vi "Alpha Transparency and Z-Order.vi"() -> ()   [LabVIEW 2011]
uses:
  <vilib>/Heliosphere Research LLC/Advanced Plotting Toolkit/Advanced Plotting Toolkit.lvlib
  <vilib>/Heliosphere Research LLC/Advanced Plotting Toolkit/api_plotting/Histogram_Automatic.vi
  <vilib>/Heliosphere Research LLC/Advanced Plotting Toolkit/api_plotting/HistogramRange.ctl
  <vilib>/Heliosphere Research LLC/Advanced Plotting Toolkit/typedefs/PlotColor.ctl
  <vilib>/Heliosphere Research LLC/Advanced Plotting Toolkit/properties/Line_Style.ctl
  <vilib>/Heliosphere Research LLC/Advanced Plotting Toolkit/properties/Line.ctl
  <vilib>/Heliosphere Research LLC/Advanced Plotting Toolkit/properties/Display.ctl
  <vilib>/Heliosphere Research LLC/Advanced Plotting Toolkit/api_plotting/HistogramProperties.ctl
  <vilib>/Heliosphere Research LLC/Advanced Plotting Toolkit/properties/Text_FontSize.ctl
  <vilib>/Heliosphere Research LLC/Advanced Plotting Toolkit/properties/Text_FontStyle.ctl
  <vilib>/Heliosphere Research LLC/Advanced Plotting Toolkit/properties/Text.ctl
  <vilib>/Heliosphere Research LLC/Advanced Plotting Toolkit/api_annotations/TextProperties.ctl
panel:
  in  "Show Text":bool
  in  "Text Z-Order":dbl
  in  "Histogram Alpha":dbl=0.6
  out "Alpha Demo":picture
  # "Alpha Transparency and Z-Order"
  # "Most plotting VIs in the tookit have a Display sub-cluster\nin the property cluster.  This allows you to adjust how the\nobjects are rendered.\n\nWhen multiple plotting VIs are called, the objects are \"stacked\"\naccording to their Z-order.  This number is automatically\nassigned by the Toolkit and keeps e.g. text in front of bars and\nlines.  You can manually adjust the Z order to force objects\nto be displayed in front of or behind other objects.  Try it\nbelow; turn the sample text on and adjust its Z-Order.\n\nNormally, objects are opaque.  However, you can enable\ntransparency using the Display.Alpha value.  This value ranges\nfrom 0 (fully transparent) to 1 (fully opaque).  Traditional\nalpha-blending is used, which can combine multiple partially-\ntransparent objects along with the plot background color.\n\nIn this example, two histogram plots are made, and their\nalpha values set to 0.6. Try changing this value and see the\nresults."
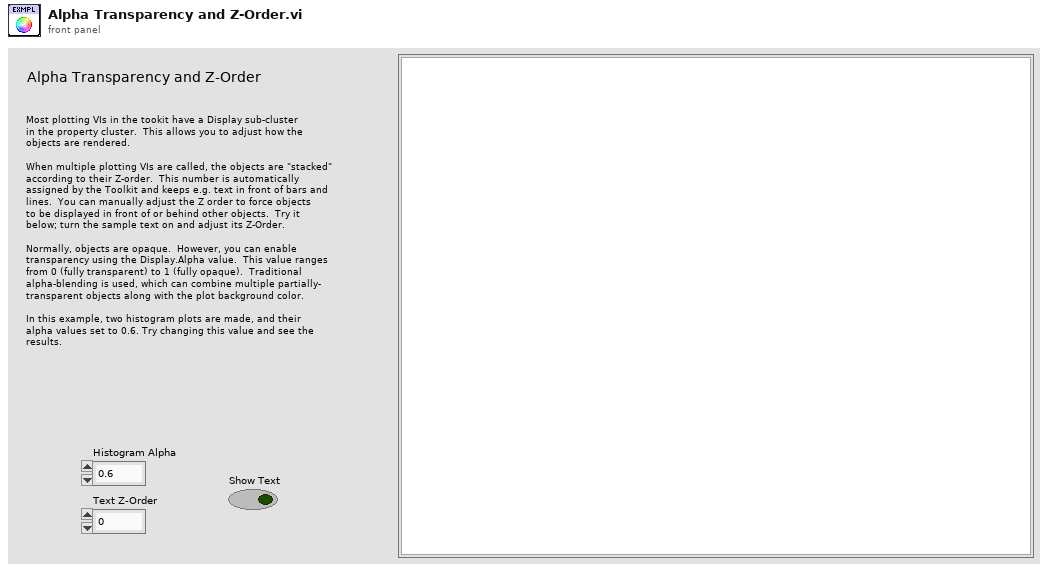
[diagram p1: front panel]
types:
  T1 = typedef "Advanced Plotting Toolkit.lvlib/TextProperties.ctl" = cluster{"Text":T2, "Display":T6}
  T2 = typedef "Advanced Plotting Toolkit.lvlib/Text.ctl" = cluster{"Color":T3, "Background Color":T3, "Font Size (points)":T4, "Font Style":T5, "Rotation Angle":dbl}
  T3 = typedef "Advanced Plotting Toolkit.lvlib/PlotColor.ctl" = u32
  T4 = typedef "Advanced Plotting Toolkit.lvlib/Text_FontSize.ctl" = i32
  T5 = typedef "Advanced Plotting Toolkit.lvlib/Text_FontStyle.ctl" = enum16{"Automatic", "Normal", "Italic", "Bold"}
  T6 = typedef "Advanced Plotting Toolkit.lvlib/Display.ctl" = cluster{"Alpha":dbl, "Z Order":dbl}
  T7 = typedef "Advanced Plotting Toolkit.lvlib/HistogramRange.ctl" = cluster{"Data Min":dbl, "Data Max":dbl}
  T8 = typedef "Advanced Plotting Toolkit.lvlib/HistogramProperties.ctl" = cluster{"Color":T3, "Cumulative":bool, "Normalize":bool, "Line":T9, "Display":T6}
  T9 = typedef "Advanced Plotting Toolkit.lvlib/Line.ctl" = cluster{"Style":T10, "Color":T3, "Width":sgl}
  T10 = typedef "Advanced Plotting Toolkit.lvlib/Line_Style.ctl" = enum16{"Automatic", "Solid", "Dashed", "Dotted", "Dash-dot", "Invisible"}
  T11 = typedef "Advanced Plotting Toolkit.lvlib/PlotID.ctl" = i32
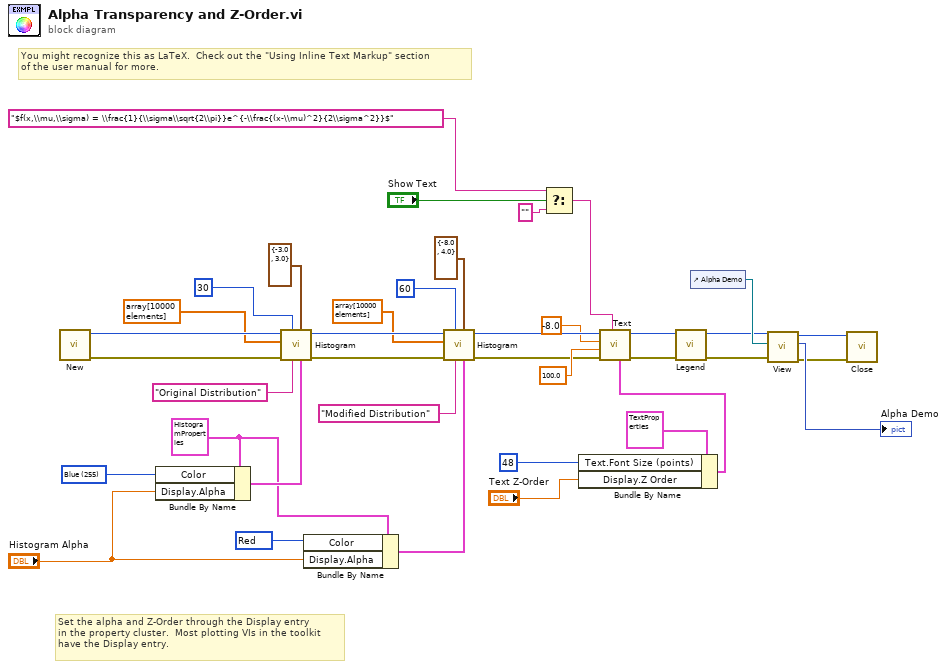
[diagram p0: block diagram]
diagram:
  w28 = T3 16711680 items=["Automatic"=2147483647, "Black"=0, "White"=16777215, "Red"=16711680, "Green"=2263842, "Blue"=255, "Cyan"=65535, "Magenta"=16711935, "Yellow"=16776960] ("Color")
  w32 = T3 255 items=["Automatic"=2147483647, "Black"=0, "White"=16777215, "Red"=16711680, "Green"=2263842, "Blue"=255, "Cyan"=65535, "Magenta"=16711935, "Yellow"=16776960] ("Color")
  w27 = T8 {"Color"=2147483647, "Cumulative"=FALSE, "Normalize"=FALSE, "Line"={"Style"=enum."Automatic", "Color"=2147483647, "Width"=nan}, "Display"={"Alpha"=nan, "Z Order"=nan}} ("Histogram Properties")
  # "You might recognize this as LaTeX.  Check out the \"Using Inline Text Markup\" section\nof the user manual for more."
  # "Set the alpha and Z-Order through the Display entry\nin the property cluster.  Most plotting VIs in the toolkit\nhave the Display entry."
  n1 = call <vilib>:"New.vi"() -> ("error out"=w11:errorcluster, "Plot ID"=w35:T11)  [unwired: 10 in]
  n2 = Bundle By Name(cluster=w27, "Color"=w32, "Display.Alpha"="Histogram Alpha") -> (w33:T8)
  n3 = call-poly <vilib>:"Histogram.vi"("Properties"=w33, "Data Range"=T7 {"Data Min"=-3.0, "Data Max"=3.0}, "Legend Title"="Original Distribution" ("String"), "Bins"=30, "error in (no error)"=w11, "Data"=dbl[] array[10000 elements] ("Gaussian noise pattern"), "Plot ID"=w35) -> ("error out"=w10:errorcluster, "Plot ID Out"=w30:T11)  [unwired: 3 in]
  n4 = Bundle By Name(cluster=w27, "Color"=w28, "Display.Alpha"="Histogram Alpha") -> (w26:T8)
  n5 = call-poly <vilib>:"Histogram.vi"("Properties"=w26, "Data Range"=T7 {"Data Min"=-8.0, "Data Max"=4.0}, "Legend Title"="Modified Distribution" ("String"), "Bins"=60, "error in (no error)"=w10, "Data"=dbl[] array[10000 elements] ("x-y"), "Plot ID"=w30) -> ("error out"=w9:errorcluster, "Plot ID Out"=w23:T11)  [unwired: 3 in]
  n6 = Select(t="$f(x,\\mu,\\sigma) = \\frac{1}{\\sigma\\sqrt{2\\pi}}e^{-\\frac{(x-\\mu)^2}{2\\sigma^2}}$" ("Text"), s="Show Text", f="" ("Text")) -> (s? t:f=w12:string)
  n7 = Bundle By Name(cluster=T1 {"Text"={"Color"=2147483647, "Background Color"=2147483647, "Font Size (points)"=0, "Font Style"=enum."Automatic", "Rotation Angle"=nan}, "Display"={"Alpha"=nan, "Z Order"=nan}} ("Text Properties"), "Text.Font Size (points)"=48, "Display.Z Order"="Text Z-Order") -> (w18:T1)
  n8 = call <vilib>:"Text.vi"("Properties"=w18, "Text"=w12, "error in (no error)"=w9, "Y Position"=100.0, "X Position"=-8.0, "Plot ID"=w23) -> ("error out"=w8:errorcluster, "Plot ID Out"=w22:T11)  [unwired: 4 in]
  n9 = call <vilib>:"Legend.vi"("error in (no error)"=w8, "Plot ID"=w22) -> ("error out"=w7:errorcluster, "Plot ID Out"=w24:T11)  [unwired: 8 in]
  n10 = control-ref of="Alpha Demo"() -> (w38:refnum<vi>)
  n11 = call <vilib>:"View.vi"("error in (no error)"=w7, "Ref for Sizing"=w38, "Plot ID"=w24) -> ("error out"=w1:errorcluster, "Picture"=→"Alpha Demo":picture, "Plot ID Out"=w36:T11)  [unwired: 6 in]
  n12 = call <vilib>:"Close.vi"("error in (no error)"=w1, "Plot ID"=w36) -> ()  [unwired: 9 in, 1 out]
